vi "SequenceDemo_dlg.vi"(8 "error in (no error)":errorcluster, 11 "NumberOfAxes":u8) -> (0 "error out":errorcluster, 2 "Sequence Paras":T1 {"End position" format="%.2f"; "Start position" format="%.2f"}, 3 "OK Out":bool)   [LabVIEW 2018]
uses:
  SequenceParam.ctl
panel:
  in  "End position":dbl[](array[numeric])=[4.0, 5.0, 6.0] format="%.2f"
  in  "Start position":dbl[](array[numeric])=[0.0, 1.0, 2.0] format="%.2f"
  in  "Number of cycles":i32=5
  in  "Cancel":bool caption="Stop"
  in  "OK":bool
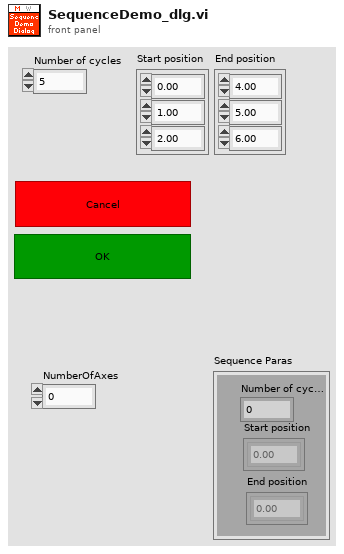
[diagram p1: front panel]
types:
  T1 = typedef "SequenceParam.ctl" = cluster{"Number of cycles":i32, "Start position":dbl[], "End position":dbl[]}
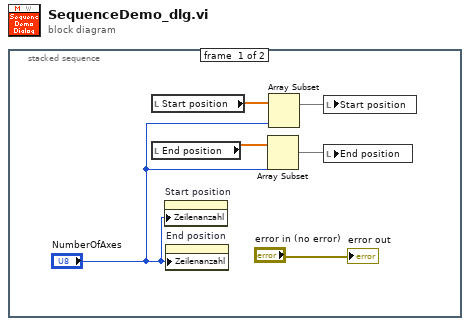
[diagram p0: block diagram]
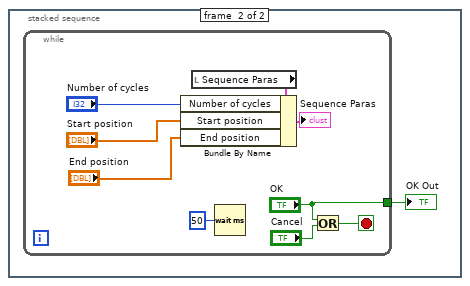
[diagram p2: hidden frame]
diagram:
  n1 = stacked-sequence {
    frame #0 {
      n2 = local read "Start position"() -> (w5:dbl[])
      n3 = local read "End position"() -> (w4:dbl[])
      n4 = property on="Start position" class="Arr (strict)"("Zeilenanzahl"="NumberOfAxes") -> ()  [unwired: 2 in, 2 out]
      n5 = property on="End position" class="Arr (strict)"("Zeilenanzahl"="NumberOfAxes") -> ()  [unwired: 2 in, 2 out]
      n6 = Array Subset(array=w4, length="NumberOfAxes") -> (w2:dbl[])  [unwired: 1 in]
      n7 = Array Subset(array=w5, length="NumberOfAxes") -> (w3:dbl[])  [unwired: 1 in]
      n8 = local write "Start position"(w3) -> ()
      n9 = local write "End position"(w2) -> ()
      "error out" <- "error in (no error)"
    }
    frame #1 {
      n10 = while {
        tunnel: ["OK"] -> w7
        stop <- w15 stop-if-true
        n11 = local read "Sequence Paras"() -> (w13:T1)
        n12 = Bundle By Name(cluster=w13, "Number of cycles"="Number of cycles", "Start position"="Start position", "End position"="End position") -> (→"Sequence Paras":T1)
        n13 = Wait (ms)(milliseconds to wait=u32 50) -> ()  [unwired: 1 out]
        n14 = Or(x="OK", y="Cancel") -> (x .or. y?=w15:bool)
      }
      "OK Out" <- w7
    }
  }
